vi "ArmLimit.vi"(9 "Extend":dbl, 10 "Lift":dbl, 11 "Rotate":dbl) -> (1 "Extend":dbl, 2 "Lift":dbl, 3 "Rotate":dbl)   [LabVIEW 2020]
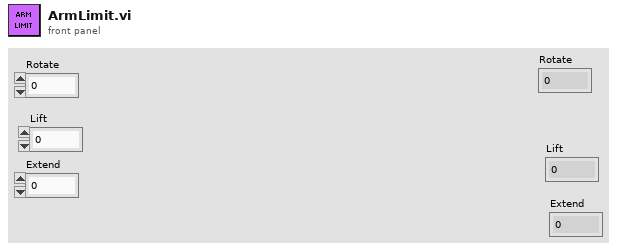
[diagram p1: front panel]
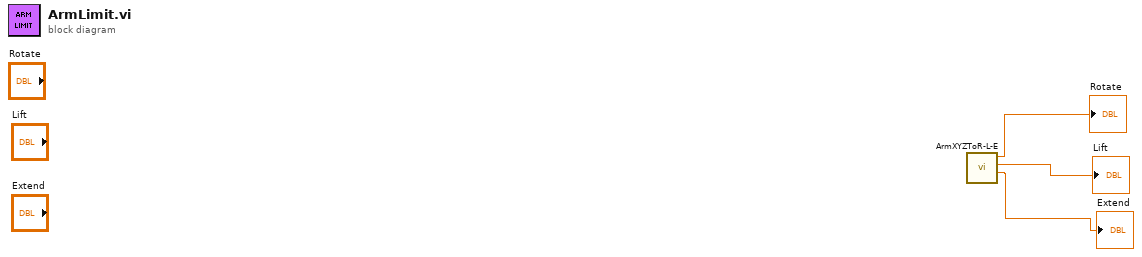
[diagram p0: block diagram]
diagram:
  n1 = call "ArmXYZToR-L-E.vi"() -> ("Extend"=→"Extend":dbl, "Lift"=→"Lift":dbl, "Rotate"=→"Rotate":dbl)  [unwired: 9 in]
